vi "State with Event.vi"() -> ()   [LabVIEW 2022 SP3]
panel:
  out "Number Display":dbl
  in  "stop":bool
  in  "Number Generate":bool
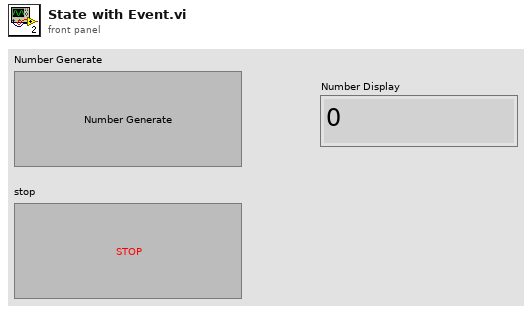
[diagram p1: front panel]
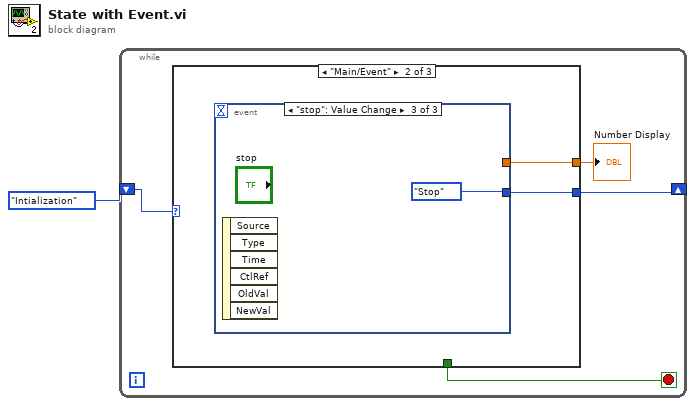
[diagram p0: block diagram]
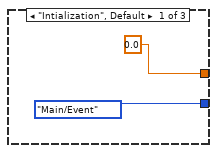
[diagram p2: hidden frame]
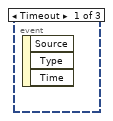
[diagram p3: hidden frame]
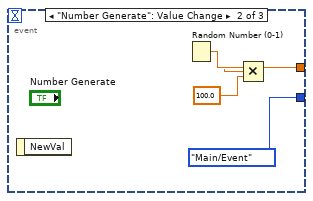
[diagram p4: hidden frame]
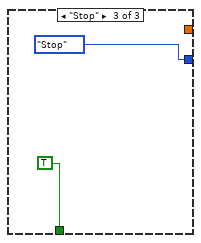
[diagram p5: hidden frame]
diagram:
  n1 = while {
    shift-right: [w4] -> _
    shift-left: enum16{"Intialization", "Main/Event", "Stop"}."Intialization" -> [w5]
    stop <- w2 stop-if-true
    n2 = case shown="\"Main/Event\"" w5 {
      tunnel: [enum16{"Intialization", "Main/Event", "Stop"}."Main/Event" w8 enum16{"Intialization", "Main/Event", "Stop"}."Stop"] -> w4
      tunnel: [0.0 w9 _] -> w3
      tunnel: [_ _ TRUE] -> w2
      frame "Intialization", Default {
      }
      frame "Main/Event" {
        n3 = event shown="[2] \"stop\": Value Change" {
          selector: _ -> [_ _ _]
          dyn-events: _ -> [_ _ _]
          timeout: _ -> [_ _ _]
          tunnel: [_ w11 _] -> w9
          tunnel: [_ enum16{"Intialization", "Main/Event", "Stop"}."Main/Event" enum16{"Intialization", "Main/Event", "Stop"}."Stop"] -> w8
          event Timeout {
            n4 = event-data() -> ()  [unwired: 1 in, 3 out]
          }
          event "Number Generate": Value Change {
            n5 = event-data() -> ()  [unwired: 1 in, 1 out]
            n6 = Random Number (0-1)() -> (number: 0 to 1=w13:dbl)
            n7 = Multiply(x=w13, y=100.0) -> (x*y=w11:dbl)
          }
          event "stop": Value Change {
            n8 = event-data() -> ()  [unwired: 1 in, 6 out]
          }
        }
      }
      frame "Stop" {
      }
    }
    "Number Display" <- w3
  }
